vi "Read Model Data.vi"(8 "error in (no error)":errorcluster, 10 "meas_timestamp in":timestamp, 11 "ChromaPowerSupplyModel in":refnum<class "ChromaPowerSupplyModel.lvclass">) -> (0 "error out":errorcluster, 2 "ICDAS2Model Data":T1[](array[typedef]), 3 "ChromaPowerSupplyModel out":refnum<class "ChromaPowerSupplyModel.lvclass">)   [LabVIEW 2018, in "AcPwrPlugins.lvlib" / "ChromaPowerSupplyModel.lvclass"]
uses:
  ChromaPowerSupplyModel.lvclass
  TypeDefs/ChromaPS_Model2ICDAS.ctl
  ChromaPowerSupplyModel.lvclass/ChromaPowerSupplyModel.ctl
  <vilib>/addons/database/_DB Variant To Data/Database Variant To Data.xnode
  Database/DatabaseBaseClass/DatabaseBaseClass.lvclass
  <vilib>/addons/database/NI_Database_API.lvlib
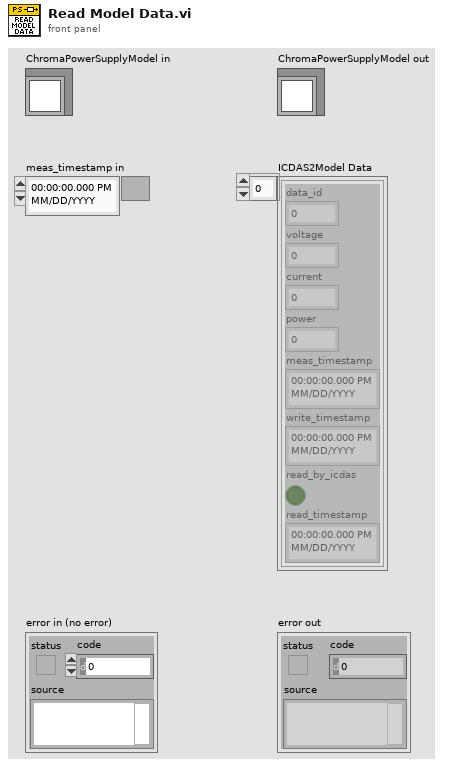
[diagram p1: front panel]
types:
  T1 = typedef "AcPwrPlugins.lvlib/ChromaPowerSupplyModel.lvclass/ChromaPS_Model2ICDAS.ctl" = cluster{"data_id":i32, "voltage":dbl, "current":dbl, "power":dbl, "meas_timestamp":timestamp, "write_timestamp":timestamp, "read_by_icdas":bool, "read_timestamp":timestamp}
  T2 = typedef "NI_Database_API.lvlib/Conn ObjectReference.ctl" = refnum<k1>
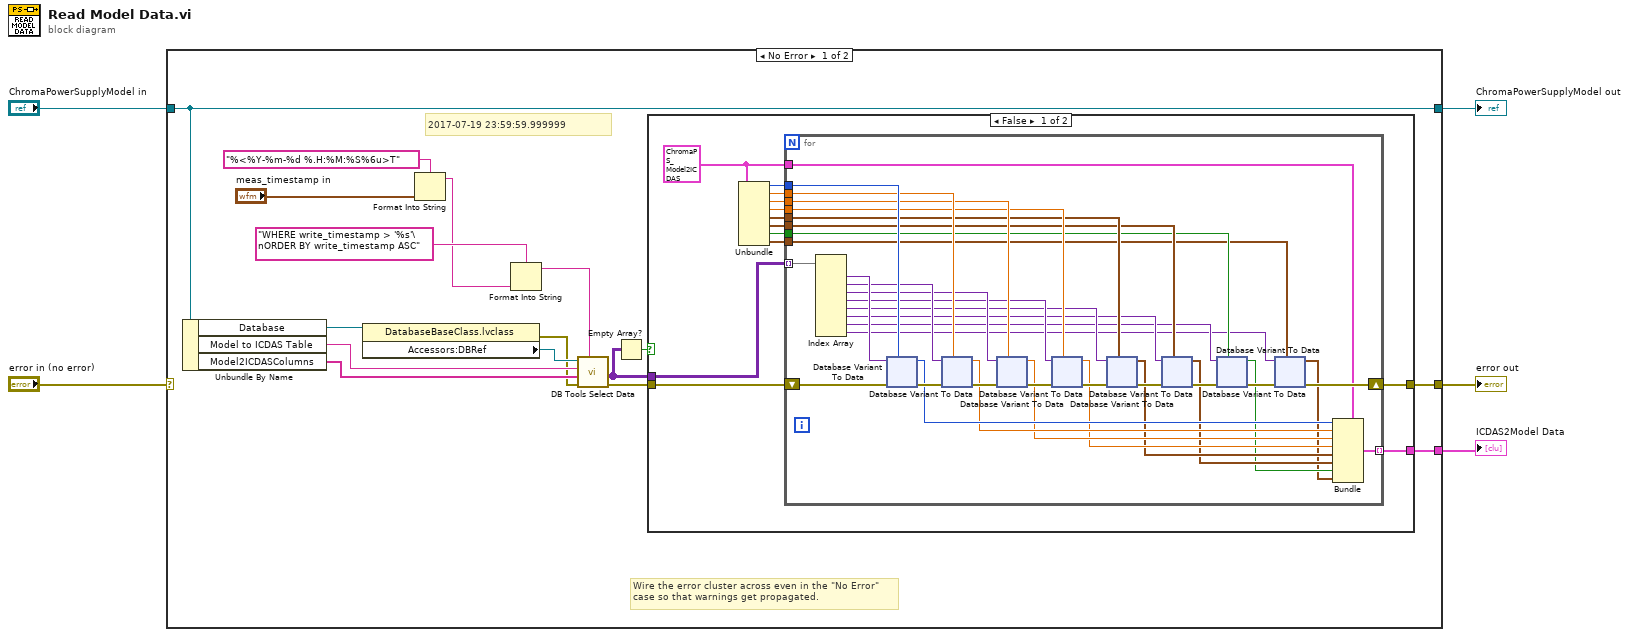
[diagram p0: block diagram]
diagram:
  n1 = case shown="No Error" "error in (no error)" {
    selector: "error in (no error)" -> [_ w368]
    tunnel: [w11 w368] -> w4
    tunnel: [w15 w367] -> w2
    tunnel: "ChromaPowerSupplyModel in" -> [w15 w367]
    tunnel: [w14 _] -> w1
    frame No Error {
      # "2017-07-19 23:59:59.999999"
      # "Wire the error cluster across even in the \"No Error\"\ncase so that warnings get propagated."
      n2 = Unbundle By Name(w15) -> ("Database"=w21:refnum<class "DatabaseBaseClass.lvclass">, "Model to ICDAS Table"=w20:string, "Model2ICDASColumns"=w18:string[])
      n3 = property class="DatabaseBaseClass.lvclass"(reference=w21) -> (error out=w17:errorcluster, "Accessors:DBRef"=w19:T2)  [unwired: 1 in, 1 out]
      n4 = Format Into String(format string="%<%Y-%m-%d %.H:%M:%S%6u>T", "meas_timestamp in") -> (resulting string=w7:string)  [unwired: 2 in, 1 out]
      n5 = Format Into String(format string="WHERE write_timestamp > '%s'\nORDER BY write_timestamp ASC" ("condition"), w7) -> (resulting string=w6:string)  [unwired: 2 in, 1 out]
      n6 = call <vilib>:"DB Tools Select Data.vi"("condition"=w6, "error in (no error)"=w17, "columns"=w18, "table"=w20, "connection reference"=w19) -> ("error out"=w16:errorcluster, "data"=w12:variant[][])  [unwired: 1 in, 1 out]
      n7 = Empty Array?(array=w12) -> (empty?=w13:bool)
      n8 = case shown="False" w13 {
        tunnel: w16 -> [w34 w366]
        tunnel: w12 -> [w33 _]
        tunnel: [w23 _] -> w14
        tunnel: [w22 w366] -> w11
        frame False {
          w24 = T1 {"data_id"=0, "voltage"=0.0, "current"=0.0, "power"=0.0, "meas_timestamp"=timestamp(0 s since 1904-01-01), "write_timestamp"=timestamp(0 s since 1904-01-01), "read_by_icdas"=FALSE, "read_timestamp"=timestamp(0 s since 1904-01-01)} ("ChromaPS_Model2ICDAS")
          n9 = Unbundle(w24) -> ("data_id"=w32:i32, "voltage"=w31:dbl, "current"=w30:dbl, "power"=w29:dbl, "meas_timestamp"=w28:timestamp, "write_timestamp"=w27:timestamp, "read_by_icdas"=w26:bool, "read_timestamp"=w25:timestamp)
          n10 = for {
            shift-right: [w54] -> w22
            shift-left: w34 -> [w70]
            tunnel: w33 -> [w64] mode=indexing
            tunnel: w32 -> [w63]
            tunnel: w31 -> [w61]
            tunnel: w30 -> [w60]
            tunnel: w29 -> [w59]
            tunnel: w28 -> [w58]
            tunnel: w27 -> [w57]
            tunnel: w26 -> [w53]
            tunnel: w25 -> [w52]
            tunnel: w24 -> [w44]
            tunnel: [w35] -> w23 mode=indexing
            n11 = Index Array(array=w64) -> (element #1=w62:variant, element #2=w51:variant, element #3=w50:variant, element #4=w49:variant, element #5=w48:variant, element #6=w47:variant, element #7=w46:variant, element #8=w45:variant)  [unwired: 8 in]
            n12 = xnode "Database Variant To Data"("database variant"=w62, "error in (no error)"=w70, "type"=w63) -> ("data"=w43:i32, "error out"=w68:errorcluster)
            n13 = xnode "Database Variant To Data"("database variant"=w51, "error in (no error)"=w68, "type"=w61) -> ("data"=w42:dbl, "error out"=w67:errorcluster)
            n14 = xnode "Database Variant To Data"("database variant"=w50, "error in (no error)"=w67, "type"=w60) -> ("data"=w41:dbl, "error out"=w66:errorcluster)
            n15 = xnode "Database Variant To Data"("database variant"=w49, "error in (no error)"=w66, "type"=w59) -> ("data"=w40:dbl, "error out"=w65:errorcluster)
            n16 = xnode "Database Variant To Data"("database variant"=w48, "error in (no error)"=w65, "type"=w58) -> ("data"=w39:timestamp, "error out"=w69:errorcluster)
            n17 = xnode "Database Variant To Data"("database variant"=w47, "error in (no error)"=w69, "type"=w57) -> ("data"=w38:timestamp, "error out"=w56:errorcluster)
            n18 = xnode "Database Variant To Data"("database variant"=w46, "error in (no error)"=w56, "type"=w53) -> ("data"=w37:bool, "error out"=w55:errorcluster)
            n19 = xnode "Database Variant To Data"("database variant"=w45, "error in (no error)"=w55, "type"=w52) -> ("data"=w36:timestamp, "error out"=w54:errorcluster)
            n20 = Bundle(cluster=w44, "data_id"=w43, "voltage"=w42, "current"=w41, "power"=w40, "meas_timestamp"=w39, "write_timestamp"=w38, "read_by_icdas"=w37, "read_timestamp"=w36) -> (w35:T1)
          }
        }
        frame True {
        }
      }
    }
    frame Error {
    }
  }
  "error out" <- w4
  "ChromaPowerSupplyModel out" <- w2
  "ICDAS2Model Data" <- w1
